vi "Read EEPROM.vi"() -> ()   [LabVIEW 2019, in "Relay-Box.lvclass"]
uses:
  Relay-Box.lvclass
  Relay-Box.lvclass/Relay-Box.ctl
  <instrlib>/FTDI/D2XX/D2XX.lvlib
panel:
  out "string":string
  out "error out":errorcluster
  in  "error in (no error)":errorcluster
  out "FT_Status out":u32(ring) items=["FT_OK", "FT_INVALID_HANDLE", "FT_DEVICE_NOT_FOUND", "FT_DEVICE_NOT_OPENED", "FT_IO_ERROR", "FT_INSUFFICIENT_RESOURCES", "FT_INVALID_PARAMETER", "FT_INVALID_BAUD_RATE", "FT_DEVICE_NOT_OPENED_FOR_ERASE", "FT_DEVICE_NOT_OPENED_FOR_WRITE", "FT_FAILED_TO_WRITE_DEVICE", "FT_EEPROM_READ_FAILED", "FT_EEPROM_WRITE_FAILED", "FT_EEPROM_ERASE_FAILED", "FT_EEPROM_NOT_PRESENT", "FT_EEPROM_NOT_PROGRAMMED", "FT_INVALID_ARGS", "FT_NOT_SUPPORTED", "FT_OTHER_ERROR"]
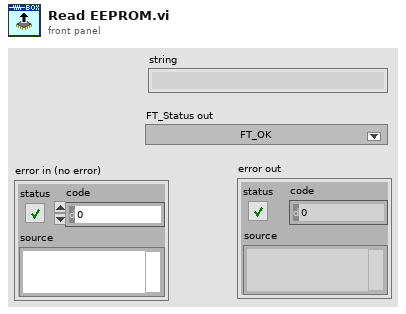
[diagram p1: front panel]
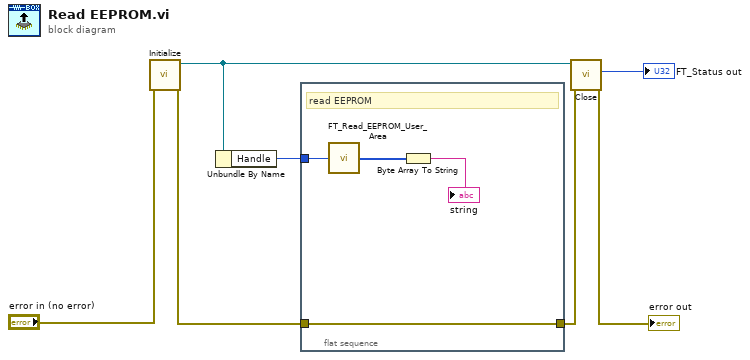
[diagram p0: block diagram]
diagram:
  n1 = call "Initialize.vi"("error in (no error)"="error in (no error)") -> ("error out"=w2:errorcluster, "Relay-Box out"=w3:refnum<class "Relay-Box.lvclass">)  [unwired: 9 in]
  n2 = Unbundle By Name(w3) -> ("Handle"=w4:u32)
  n3 = flat-sequence {
    tunnel: [w11] -> w6
    tunnel: w2 -> [w11]
    tunnel: w4 -> [w10]
    frame #0 {
      # "read EEPROM"
      n4 = call <instrlib>:"FT_Read_EEPROM_User_Area.vi"("Handle"=w10) -> ("User Area Data"=w9:u8[])  [unwired: 2 out]
      n5 = Byte Array To String(unsigned byte array=w9) -> (string=→"string":string)
    }
  }
  n6 = call "Close.vi"("error in (no error)"=w6, "Relay-Box in"=w3) -> ("error out"=→"error out":errorcluster, "FT_Status"=→"FT_Status out":u32)  [unwired: 7 in, 1 out]
